vi "Vision Processing.vi"(4 "error in (no error)":errorcluster, 7 "Image Size":T3=enum."320x240") -> ()   [LabVIEW 2018]
doc: "This VI runs in parallel to other tasks. It gets images from the camera, processes them for color or shape and use that information to affect robot behavior."
uses:
  <vilib>/Rock Robotics/WPI/Camera/WPI_CameraImageSize.ctl
  <vilib>/Rock Robotics/WPI/Camera/WPI_CameraExposure Values.ctl
  <vilib>/Rock Robotics/WPI/Camera/WPI_CameraWhite Balance Values.ctl
  <vilib>/Rock Robotics/WPI/Camera/WPI_CameraFrameRate.ctl
  Robot Global Data.vi
panel:
  in  "White Balance":T1
  in  "Color Temp (K)":dbl format="%#_13g"
  in  "Exposure (%)":dbl=50.0
  in  "Exposure":T2
  in  "Force":bool
  in  "Brightness":i32=50 min=0 max=100
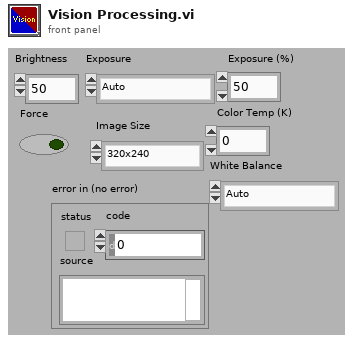
[diagram p1: front panel]
types:
  T1 = typedef "WPI_CameraWhite Balance Values.ctl" = enum16{"Auto", "Fixed indoor", "Fixed outdoor 1", "Fixed outdoor 2", "Fixed fluorescent 1", "Fixed fluorescent 2", "Hold current", "Custom"}
  T2 = typedef "WPI_CameraExposure Values.ctl" = enum16{"Auto", "Flicker-free 50 Hz", "Flicker-free 60 Hz", "Hold current", "Custom"}
  T3 = typedef "WPI_CameraImageSize.ctl" = enum16{"640x480", "320x240", "160x120", "Custom"}
  T4 = typedef "WPI_CameraFrameRate.ctl" = u32
  T5 = typedef "Image Type" = u32
  T6 = typedef "WPI_CameraDevRef.ctl" = cluster{"Camera Address":string, "CameraStatus":errorcluster}
  T7 = typedef "IMAQ Image.ctl" = refnum<image>
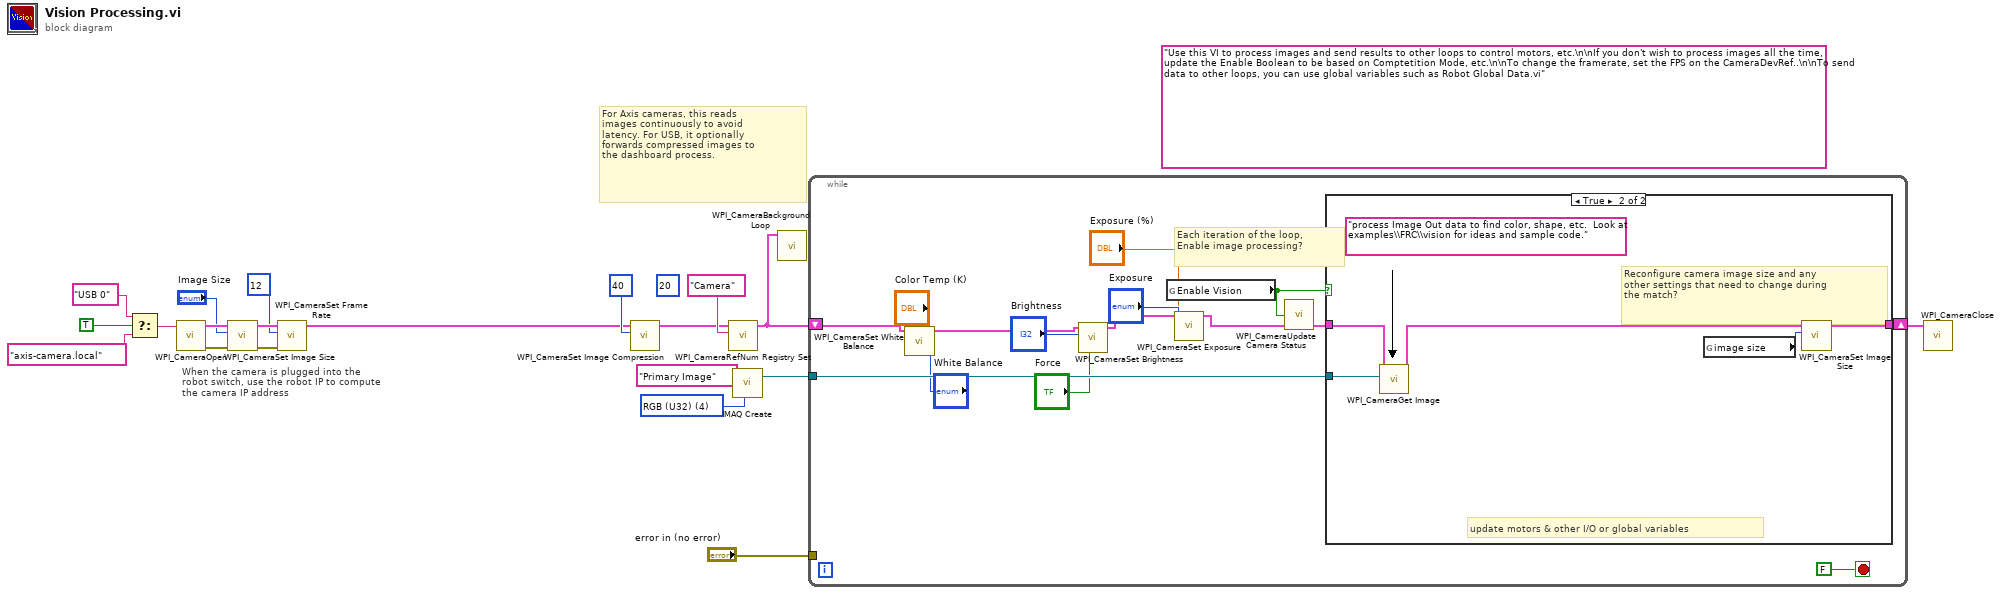
[diagram p0: block diagram]
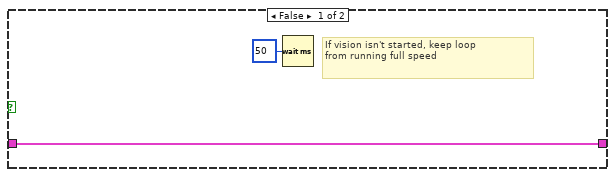
[diagram p2: hidden frame]
diagram:
  (unwired) 20 ("Brightness")
  (unwired) "Use this VI to process images and send results to other loops to control motors, etc.\n\nIf you don't wish to process images all the time, update the Enable Boolean to be based on Comptetition Mode, etc.\n\nTo change the framerate, set the FPS on the CameraDevRef..\n\nTo send data to other loops, you can use global variables such as Robot Global Data.vi"
  w20 = T5 4 items=["Grayscale (U8)", "Grayscale (I16)", "Grayscale (SGL)", "Complex (CSG)", "RGB (U32)", "HSL (U32)", "RGB (U64)"] ("Image Type")
  # "When the camera is plugged into the\nrobot switch, use the robot IP to compute\nthe camera IP address"
  # "For Axis cameras, this reads\nimages continuously to avoid\nlatency. For USB, it optionally\nforwards compressed images to\nthe dashboard process."
  n1 = Select(t="USB 0" ("format string"), s=TRUE ("dot notation? (F)"), f="axis-camera.local" ("format string")) -> (s? t:f=w4:string)
  n2 = call <vilib>:"WPI_CameraOpen.vi"("Camera Address"=w4) -> ("error out"=w13:errorcluster, "CameraDevRef"=w14:T6)  [unwired: 1 in, 8 out]
  n3 = call <vilib>:"WPI_CameraSet Image Size.vi"("error in (no error)"=w13, "Image Size"="Image Size", "CameraDevRef"=w14) -> ("error out"=w12:errorcluster, "CameraDevRef Out"=w15:T6)  [unwired: 1 in, 6 out]
  n4 = call <vilib>:"WPI_CameraSet Frame Rate.vi"("error in (no error)"=w12, "Frame Rate (fps)"=T4 12, "CameraDevRef"=w15) -> ("CameraDevRef Out"=w1:T6)  [unwired: 8 out]
  n5 = call <vilib>:"WPI_CameraSet Image Compression.vi"("Compression"=40, "CameraDevRef"=w1) -> ("CameraDevRef Out"=w2:T6)  [unwired: 1 in, 8 out]
  n6 = call <vilib>:"WPI_CameraRefNum Registry Set.vi"("refnum name"="Camera", "CameraDevRef"=w2) -> ("CameraDevRef"=w10:T6)  [unwired: 2 in, 7 out]
  n7 = call "IMAQ Create"("Image Name"="Primary Image", "Image Type"=w20) -> ("New Image"=w18:T7)  [unwired: 2 in, 2 out]
  n8 = call <vilib>:"WPI_CameraBackground Loop.vi"("CameraDevRef"=w10) -> ()  [unwired: 11 in]
  n9 = while {
    shift-right: [w34] -> w8
    shift-left: w10 -> [w27]
    tunnel: w18 -> [w33]
    tunnel: "error in (no error)" -> [_]
    stop <- FALSE stop-if-true
    # "Each iteration of the loop,\nEnable image processing?"
    n10 = call <vilib>:"WPI_CameraSet White Balance.vi"("Color Temp (K)"="Color Temp (K)", "White Balance"="White Balance", "CameraDevRef"=w27) -> ("CameraDevRef Out"=w28:T6)  [unwired: 7 in, 1 out]
    n11 = call <vilib>:"WPI_CameraSet Brightness.vi"("Force"="Force", "Brightness"="Brightness", "CameraDevRef"=w28) -> ("CameraDevRef Out"=w29:T6)  [unwired: 7 in, 1 out]
    n12 = global read "Robot Global Data.vi" "Enable Vision"() -> (w31:bool)
    n13 = call <vilib>:"WPI_CameraSet Exposure.vi"("Exposure (%)"="Exposure (%)", "Exposure"="Exposure", "CameraDevRef"=w29) -> ("CameraDevRef Out"=w30:T6)  [unwired: 7 in, 1 out]
    n14 = call <vilib>:"WPI_CameraUpdate Camera Status.vi"("CameraDevRef In"=w30, "Enable Vision"=w31) -> ("CameraDevRef Out"=w32:T6)  [unwired: 3 in]
    n15 = case shown="True" w31 {
      tunnel: w33 -> [_ w41]
      tunnel: [w37 w42] -> w34
      tunnel: w32 -> [w37 w39]
      frame False {
        # "If vision isn't started, keep loop\nfrom running full speed"
        n16 = Wait (ms)(milliseconds to wait=u32 50) -> ()  [unwired: 1 out]
      }
      frame True {
        (unwired) "process Image Out data to find color, shape, etc.  Look at examples\\FRC\\vision for ideas and sample code."
        # "update motors & other I/O or global variables"
        # "Reconfigure camera image size and any\nother settings that need to change during\nthe match?"
        n17 = call <vilib>:"WPI_CameraGet Image.vi"("Image"=w41, "CameraDevRef"=w39) -> ("CameraDevRef Out"=w38:T6)  [unwired: 1 in, 8 out]
        n18 = global read "Robot Global Data.vi" "image size"() -> (w40:T3)
        n19 = call <vilib>:"WPI_CameraSet Image Size.vi"("Image Size"=w40, "CameraDevRef"=w38) -> ("CameraDevRef Out"=w42:T6)  [unwired: 2 in, 7 out]
      }
    }
  }
  n20 = call <vilib>:"WPI_CameraClose.vi"("CameraDevRef"=w8) -> ()  [unwired: 1 in, 10 out]
